vi "例10.5  利用底层函数连续采集图像.vi"() -> ()   [LabVIEW 2017]
doc: "The Grab VI acquires images continuously and displays the images in an image control using low-level acquisition VIs. A grab is appropriate for high-speed applications in which you need to process only one image at a time."
uses:
  <vilib>/userdefined/High Color/IMAQdx.ctl
  <vilib>/vision/driver/IMAQdx.llb/IMAQdx Acquisition Mode.ctl
  <vilib>/vision/driver/IMAQdx.llb/IMAQdx Buffer Number Mode.ctl
  <vilib>/vision/driver/NI_Vision_Acquisition_Software.lvlib
panel:
  in  "Camera Name":T1
  out "Buffer Number":u32
  out "Image":T2(plugin-control)
  in  "stop":bool
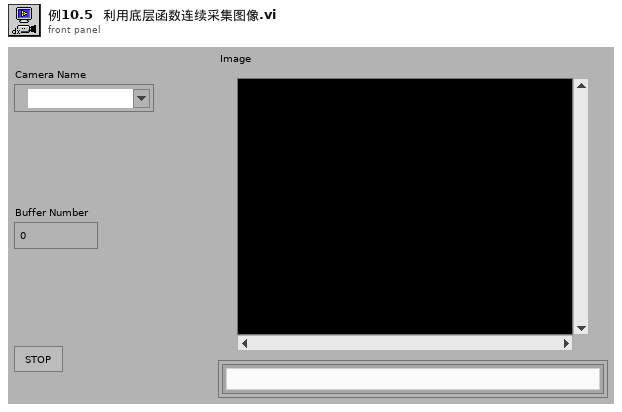
[diagram p1: front panel]
types:
  T1 = typedef "IMAQdx.ctl" = refnum<k21>
  T2 = typedef "IMAQ Image.ctl" = refnum<image>
  T3 = typedef "NI_Vision_Acquisition_Software.lvlib/IMAQdx Acquisition Mode.ctl" = enum32{"One Shot", "Continuous"}
  T4 = typedef "NI_Vision_Acquisition_Software.lvlib/IMAQdx Buffer Number Mode.ctl" = enum32{"Next", "Last", "Buffer Number", "Every", "Last New"}
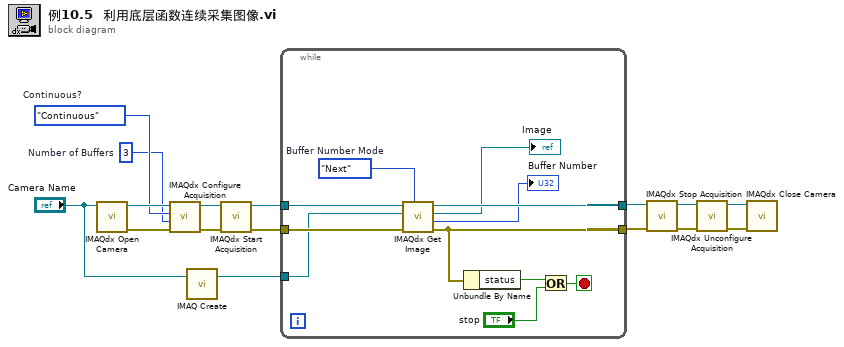
[diagram p0: block diagram]
diagram:
  w7 = u32 3  # Number of Buffers
  w8 = IMAQdx_Acquisition_Mode."Continuous"  # Continuous?
  n1 = call <vilib>:"IMAQdx Open Camera.vi"("Session In"="Camera Name") -> ("error out"=w11:errorcluster, "Session Out"=w14:T1)  [unwired: 2 in, 7 out]
  n2 = call <vilib>:"IMAQdx Configure Acquisition.vi"("error in"=w11, "Number of Buffers"=w7, "Continuous?"=w8, "Session In"=w14) -> ("error out"=w10:errorcluster, "Session Out"=w13:T1)  [unwired: 6 out]
  n3 = call "IMAQ Create"("Image Name"="Camera Name") -> ("New Image"=w16:T2)  [unwired: 3 in, 2 out]
  n4 = call <vilib>:"IMAQdx Start Acquisition.vi"("error in"=w10, "Session In"=w13) -> ("error out"=w9:errorcluster, "Session Out"=w12:T1)  [unwired: 8 out]
  n5 = while {
    tunnel: [w21] -> w5
    tunnel: w9 -> [w23]
    tunnel: w12 -> [w24]
    tunnel: [w20] -> w6
    tunnel: w16 -> [w22]
    stop <- w27 stop-if-true
    w17 = IMAQdx_Buffer_Number_Mode."Next"  # Buffer Number Mode
    n6 = call <vilib>:"IMAQdx Get Image.vi"("Buffer Number Mode (Next)"=w17, "error in"=w23, "Image In"=w22, "Session In"=w24) -> ("error out"=w20:errorcluster, "Buffer Number Out"=→"Buffer Number":u32, "Image Out"=→"Image":T2, "Session Out"=w21:T1)  [unwired: 1 in, 3 out]
    n7 = Unbundle By Name(w20) -> ("status"=w26:bool)
    n8 = Or(x=w26, y="stop") -> (x .or. y?=w27:bool)
  }
  n9 = call <vilib>:"IMAQdx Stop Acquisition.vi"("error in"=w6, "Session In"=w5) -> ("error out"=w1:errorcluster, "Session Out"=w2:T1)  [unwired: 8 out]
  n10 = call <vilib>:"IMAQdx Unconfigure Acquisition.vi"("error in"=w1, "Session In"=w2) -> ("error out"=w4:errorcluster, "Session Out"=w3:T1)  [unwired: 8 out]
  n11 = call <vilib>:"IMAQdx Close Camera.vi"("error in"=w4, "Session In"=w3) -> ()  [unwired: 10 out]
